vi "Camera Set.vi"(1 "Front Camera In":T1) -> (0 "Front Camera Out":T1)   [LabVIEW 2013]
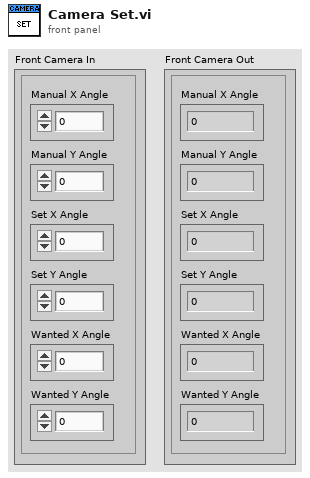
[diagram p1: front panel]
types:
  T1 = cluster{"Manual X Angle":dbl, "Manual Y Angle ":dbl, "Set X Angle":dbl, "Set Y Angle ":dbl, "Wanted X Angle":dbl, "Wanted Y Angle  ":dbl}
  T2 = typedef "WPI_ServoDeviceRef.ctl" = cluster{"DeviceStatus":errorcluster, "Digital Module":T3, "PWM Channel":T4, "DeadBand":T5}
  T3 = typedef "FPGA_TypedefDigitalModule.ctl" = enum16{"Digital Module 1", "Digital Module 2"}
  T4 = typedef "FPGA_DIOPWMChannel.ctl" = enum8{"PWM 1", "PWM 2", "PWM 3", "PWM 4", "PWM 5", "PWM 6", "PWM 7", "PWM 8", "PWM 9", "PWM 10", "Invalid"}
  T5 = typedef "WPI_PWMDeadband.ctl" = cluster{"Name":string, "maxPositivePwm":i32, "minPositivePwm":i32, "centerPwm":i32, "maxNegativePwm":i32, "minNegativePwm":i32, "angularRange":u16}
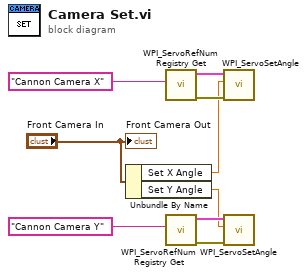
[diagram p0: block diagram]
diagram:
  n1 = Unbundle By Name("Front Camera In") -> ("Set X Angle"=w3:dbl, "Set Y Angle"=w2:dbl)
  n2 = call <vilib>:"WPI_ServoRefNum Registry Get.vi"("refnum name"="Cannon Camera X") -> ("error out"=w7:errorcluster, "ServoDeviceRef"=w6:T2)  [unwired: 9 in]
  n3 = call <vilib>:"WPI_ServoRefNum Registry Get.vi"("refnum name"="Cannon Camera Y") -> ("error out"=w4:errorcluster, "ServoDeviceRef"=w5:T2)  [unwired: 9 in]
  n4 = call <vilib>:"WPI_ServoSetAngle.vi"("error in (no error)"=w7, "Angle"=w3, "ServoDeviceRef"=w6) -> ()  [unwired: 7 in, 2 out]
  n5 = call <vilib>:"WPI_ServoSetAngle.vi"("error in (no error)"=w4, "Angle"=w2, "ServoDeviceRef"=w5) -> ()  [unwired: 7 in, 2 out]
  "Front Camera Out" <- "Front Camera In"
